vi "SetBitfiledValue(I32).vi"(8 "error in (no error)":errorcluster, 9 "bitfield value":i32, 10 "bitfield caps":T1={"offset"=0, "size"=0, "signed?"=TRUE}, 11 "original value":u64 format="%.0x") -> (0 "error out":errorcluster, 3 "update value":u64 format="%.0x")   [LabVIEW 2015, in "Bitfield.lvlib"]
uses:
  Bitfield.lvlib
  BitfieldCaps.ctl
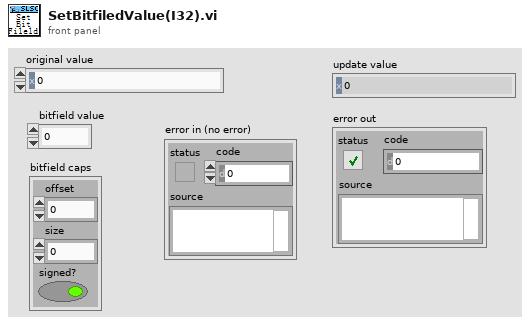
[diagram p1: front panel]
types:
  T1 = typedef "Bitfield.lvlib/BitfieldCaps.ctl" = cluster{"offset":i32, "size":i32, "signed?":bool}
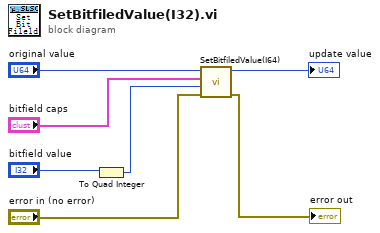
[diagram p0: block diagram]
diagram:
  n1 = To Quad Integer(1:"bitfield value") -> (0:w4:i64)
  n2 = call "SetBitfiledValue(I64).vi"("error in (no error)"="error in (no error)", "bitfield value"=w4, "bitfield caps"="bitfield caps", "original value"="original value") -> ("error out"=→"error out":errorcluster, "update value"=→"update value":u64)  [unwired: 6 in]
